vi "GEN40-38-LAN Read System Error.vi"(8 "error in (no error)":errorcluster, 11 "Resource":refnum<visa-resource-name>) -> (0 "error out":errorcluster)   [LabVIEW 2018, in "GEN40-38-LAN.lvlib" / "GEN40-38-LAN.lvclass"]
doc: "This VI is used to inquire for error messages."
uses:
  GEN40-38-LAN.lvclass
  Custom Controls/Error.ctl
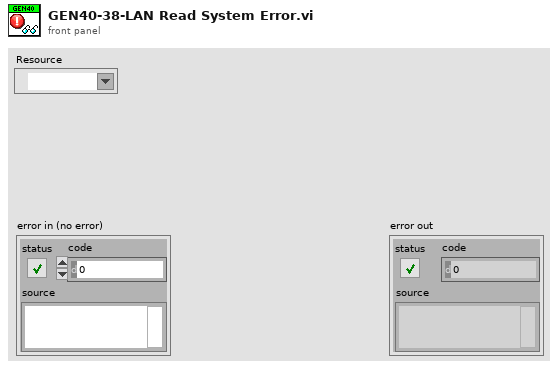
[diagram p1: front panel]
types:
  T1 = typedef "GEN40-38-LAN.lvlib/GEN40-38-LAN.lvclass/Error.ctl" = cluster{"Error Number":i32, "Error Description":string}
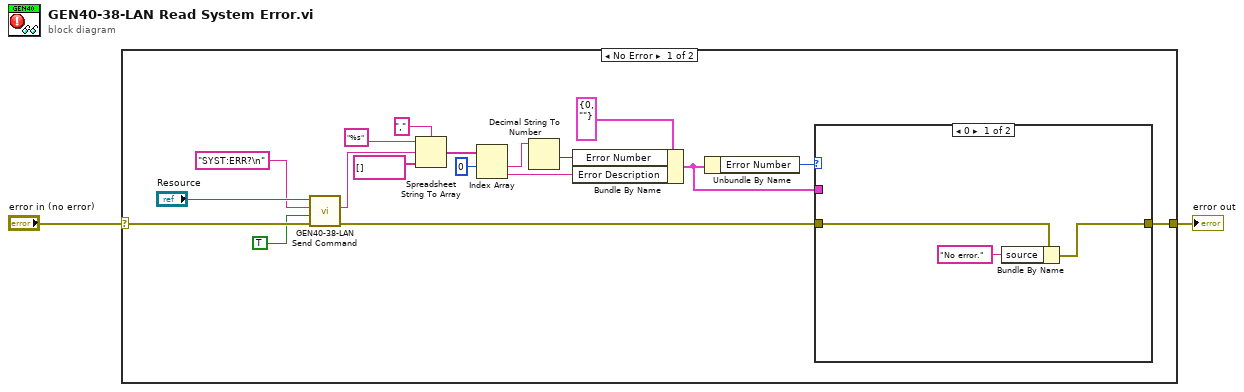
[diagram p0: block diagram]
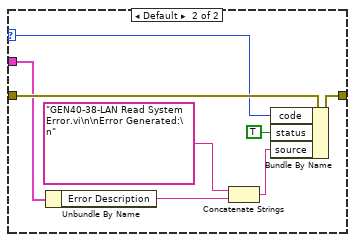
[diagram p2: hidden frame]
diagram:
  n1 = case shown="No Error" "error in (no error)" {
    selector: "error in (no error)" -> [w20 w32]
    tunnel: [w4 w32] -> w1
    frame No Error {
      n2 = call "GEN40-38-LAN Send Command.vi"("error in (no error)"=w20, "Wait for Response?"=TRUE, "Command"="SYST:ERR?\n", "VISA resource name"="Resource") -> ("error out"=w5:errorcluster, "Response"=w16:string)  [unwired: 5 in, 1 out]
      n3 = Spreadsheet String To Array(delimiter (Tab)=",", format string="%s", spreadsheet string=w16, array type (2D Dbl)=string[] []) -> (array=w12:string[])
      n4 = Index Array(array=w12, index #1=0 ("index")) -> (element #1=w10:string, element #2=w7:string)  [unwired: 1 in]
      n5 = Decimal String To Number(string=w10) -> (number=w8:i32)  [unwired: 2 in, 1 out]
      n6 = Bundle By Name(cluster=T1 {"Error Number"=0, "Error Description"=""} ("Error"), "Error Number"=w8, "Error Description"=w7) -> (w3:T1)
      n7 = Unbundle By Name(w3) -> ("Error Number"=w6:i32)
      n8 = case shown="0" w6 {
        selector: w6 -> [_ w29]
        tunnel: w5 -> [w23 w31]
        tunnel: [w22 w30] -> w4
        tunnel: w3 -> [_ w27]
        frame 0 {
          n9 = Bundle By Name(cluster=w23, "source"="No error.") -> (w22:errorcluster)
        }
        frame Default {
          n10 = Unbundle By Name(w27) -> ("Error Description"=w25:string)
          n11 = Concatenate Strings("GEN40-38-LAN Read System Error.vi\n\nError Generated:\n", w25) -> (w24:string)
          n12 = Bundle By Name(cluster=w31, "code"=w29, "status"=TRUE, "source"=w24) -> (w30:errorcluster)
        }
      }
    }
    frame Error {
    }
  }
  "error out" <- w1
